vi "Client.vi"() -> ()   [LabVIEW 2020]
uses:
  a41637b0-0f6f-4607-8673-2da23fb875f5.vi
  023a8f85-4b7b-40f0-a20a-f2dbd2322bb8.vi
  1a45ab37-82d9-4cb7-831c-46628b84d04d.vi
  8694ebda-01c4-44d9-a333-9253c2682bc0.vi
  a41637b0-0f6f-4607-8673-2da23fb875f5.vi/078ba1a1-d6bd-49b2-9c2f-e1fe39765f23.vi
  023a8f85-4b7b-40f0-a20a-f2dbd2322bb8.vi/078ba1a1-d6bd-49b2-9c2f-e1fe39765f23.vi
  1a45ab37-82d9-4cb7-831c-46628b84d04d.vi/015711cd-28da-455e-9e29-9088517d27fc.vi
  8694ebda-01c4-44d9-a333-9253c2682bc0.vi/015711cd-28da-455e-9e29-9088517d27fc.vi
  a41637b0-0f6f-4607-8673-2da23fb875f5.vi/078ba1a1-d6bd-49b2-9c2f-e1fe39765f23.vi/75f876d2-1979-4592-bbf3-d7f33a3f3770.vi
  023a8f85-4b7b-40f0-a20a-f2dbd2322bb8.vi/078ba1a1-d6bd-49b2-9c2f-e1fe39765f23.vi/75f876d2-1979-4592-bbf3-d7f33a3f3770.vi
  1a45ab37-82d9-4cb7-831c-46628b84d04d.vi/015711cd-28da-455e-9e29-9088517d27fc.vi/97430266-bf22-4483-8d6f-10177da47bcd.vi
  8694ebda-01c4-44d9-a333-9253c2682bc0.vi/015711cd-28da-455e-9e29-9088517d27fc.vi/97430266-bf22-4483-8d6f-10177da47bcd.vi
  source/Client/Client/Get Value.vi
  source/Get Library Path.vi
  <vilib>/Utility/error.llb/Error Cluster From Error Code.vi
  source/Client/Client/Put Value.vi
  source/Value/Value/Value.lvclass
  source/Client/Client.lvlib
  source/Client/Client/Client.lvclass
panel:
  in  "stop":bool
  in  "Value":dbl
  in  "Increment":bool
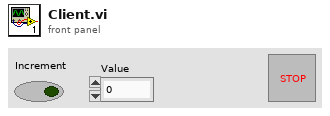
[diagram p1: front panel]
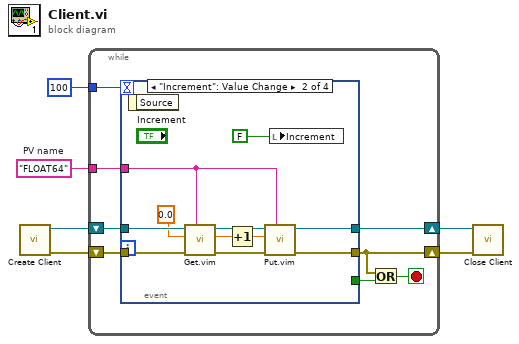
[diagram p0: block diagram]
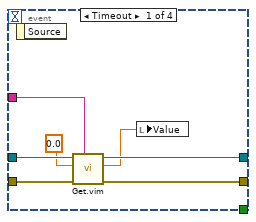
[diagram p2: hidden frame]
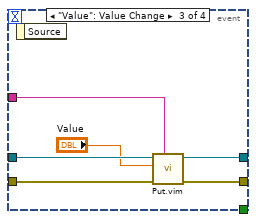
[diagram p3: hidden frame]
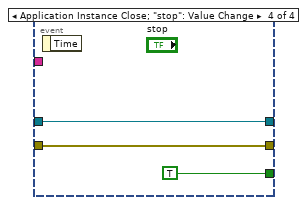
[diagram p4: hidden frame]
diagram:
  w6 = "FLOAT64"  # PV name
  n1 = call "Create Client.vi"() -> ("error out"=w2:errorcluster, "Client out"=w3:refnum<class "Client.lvclass">)  [unwired: 10 in]
  n2 = while {
    tunnel: w6 -> [w13]
    shift-right: [w11] -> w5
    shift-left: w3 -> [w12]
    shift-right: [w8] -> w4
    shift-left: w2 -> [w14]
    tunnel: 100 ("Numeric") -> [w7]
    stop <- w9 stop-if-true
    n3 = event shown="[1] \"Increment\": Value Change" {
      selector: _ -> [_ _ _ _]
      dyn-events: _ -> [_ _ _ _]
      timeout: w7 -> [_ _ _ _]
      tunnel: w14 -> [w20 w30 w38 w40]
      tunnel: w13 -> [w17 w31 w33 _]
      tunnel: w12 -> [w21 w29 w35 w39]
      tunnel: [w19 w23 w37 w40] -> w8
      tunnel: [w18 w24 w36 w39] -> w11
      tunnel: [_ _ _ TRUE] -> w10
      event Timeout {
        n4 = event-data() -> ()  [unwired: 1 in, 1 out]
        n5 = call "Get.vim"("PV name"=w17, "error in"=w20, "default"=0.0, "Client in"=w21) -> ("error out"=w19:errorcluster, "value"=w15:dbl, "Client out"=w18:refnum<class "Client.lvclass">)  [unwired: 5 in]
        n6 = local write "Value"(w15) -> ()
      }
      event "Increment": Value Change {
        n7 = event-data() -> ()  [unwired: 1 in, 1 out]
        n8 = call "Get.vim"("PV name"=w31, "error in"=w30, "default"=0.0, "Client in"=w29) -> ("error out"=w26:errorcluster, "value"=w27:dbl, "Client out"=w25:refnum<class "Client.lvclass">)  [unwired: 5 in]
        n9 = Increment(x=w27) -> (x+1=w22:dbl)
        n10 = call "Put.vim"("PV name"=w31, "error in"=w26, "value in"=w22, "Client in"=w25) -> ("error out"=w23:errorcluster, "Client out"=w24:refnum<class "Client.lvclass">)  [unwired: 5 in, 1 out]
        n11 = local write "Increment"(FALSE ("Increment")) -> ()
      }
      event "Value": Value Change {
        n12 = event-data() -> ()  [unwired: 1 in, 1 out]
        n13 = call "Put.vim"("PV name"=w33, "error in"=w38, "value in"="Value", "Client in"=w35) -> ("error out"=w37:errorcluster, "Client out"=w36:refnum<class "Client.lvclass">)  [unwired: 5 in, 1 out]
      }
      event Application Instance Close; "stop": Value Change {
        n14 = event-data() -> ()  [unwired: 1 in, 1 out]
      }
    }
    n15 = Or(x=w8, y=w10) -> (x .or. y?=w9:bool)
  }
  n16 = call "Close Client.vi"("error in (no error)"=w4, "Client in"=w5) -> ()  [unwired: 9 in, 1 out]
